vi "render.vi"(6 "Numeric":i32, 9 "origin":cluster{"left":i16, "top":i16}, 10 "new picture in":picture, 11 "map":i8[][][](array[numeric])) -> (3 "new picture out":picture)   [LabVIEW 2025]
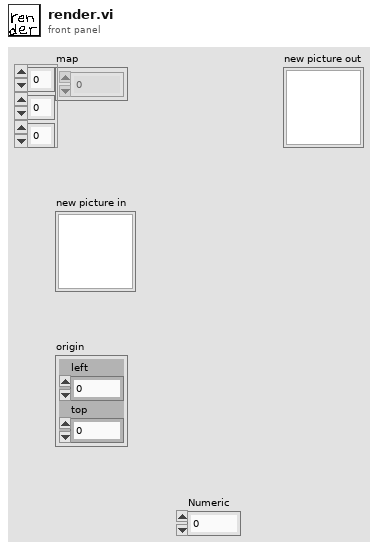
[diagram p1: front panel]
types:
  T1 = enum16{"User-specified Font", "Application Font", "System Font", "Dialog Font"}
  T2 = cluster{"Font Name:":string, "Size":i16, "Strikeout?":bool, "Italic?":bool, "Underline?":bool, "Outline?":bool, "Shadow?":bool, "Bold?":bool}
  T3 = cluster{"left":i16, "top":i16, "right":i16, "bottom":i16}
  T4 = typedef "imagedata.ctl" = cluster{"image type":i32, "image depth":i32, "image":u8[], "mask":u8[], "colors":u32[], "Rectangle":cluster{"left":i16, "top":i16, "right":i16, "bottom":i16}}
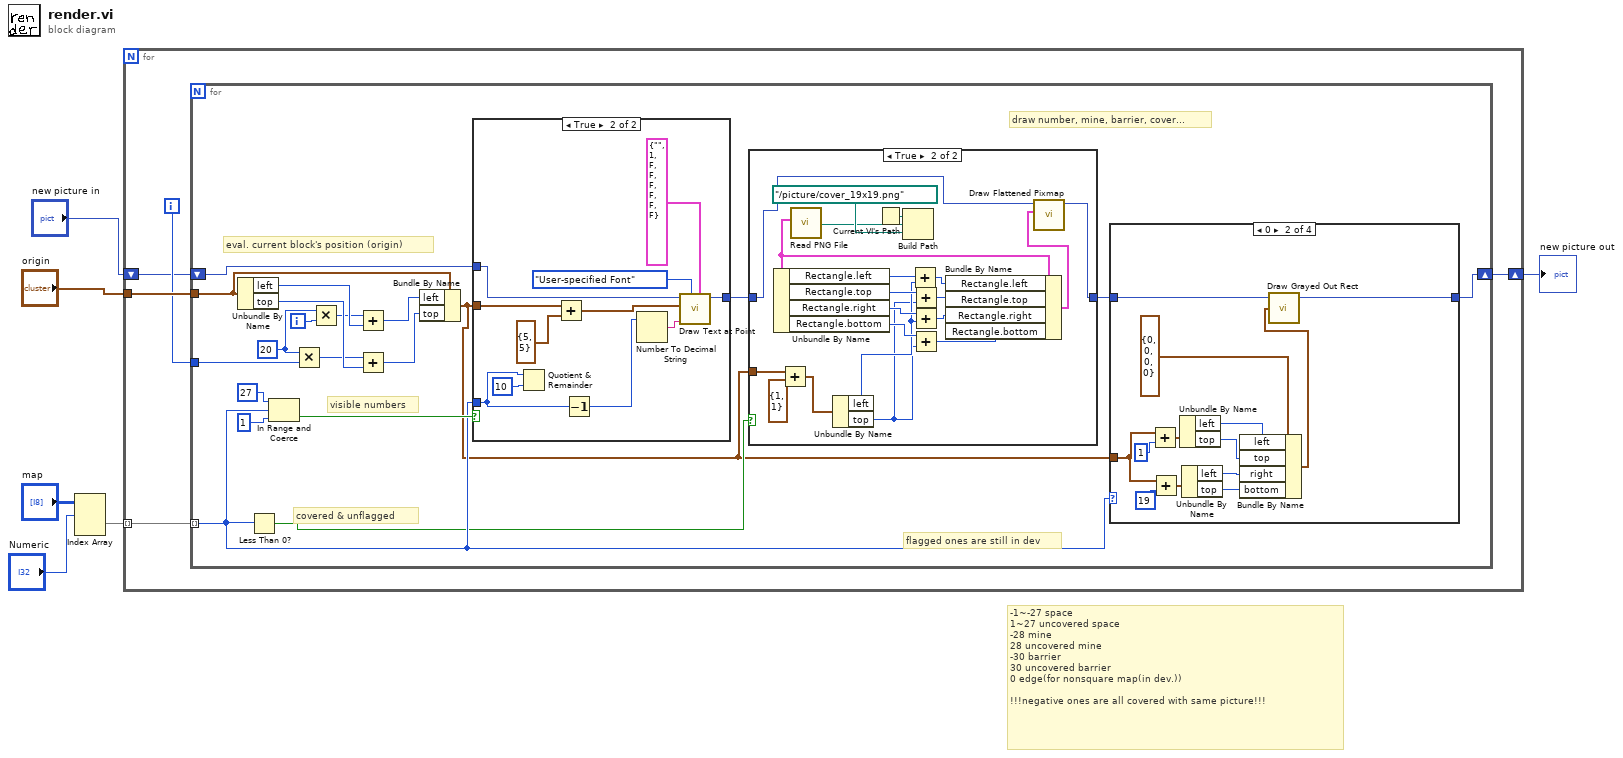
[diagram p0: block diagram]
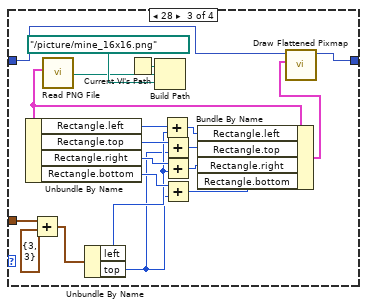
[diagram p5: hidden frame]
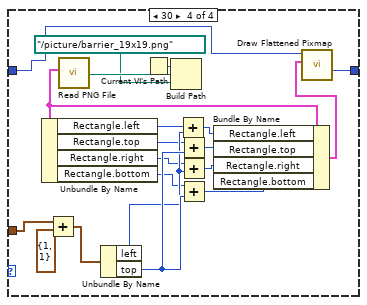
[diagram p6: hidden frame]
diagram:
  # "-1~-27 space\n1~27 uncovered space\n-28 mine\n28 uncovered mine\n-30 barrier\n30 uncovered barrier\n0 edge(for nonsquare map(in dev.))\n\n!!!negative ones are all covered with same picture!!!"
  n1 = Index Array(array="map", index (dim 0)="Numeric") -> (element=w3:i8[][])  [unwired: 2 in]
  n2 = for {
    tunnel: w3 -> [w11] mode=indexing
    tunnel: "origin" -> [w10]
    shift-right: [w7] -> w6
    shift-left: "new picture in" -> [w8]
    i -> [w9]
    n3 = for {
      tunnel: w11 -> [w14] mode=indexing
      tunnel: w10 -> [w20]
      tunnel: w9 -> [w30]
      shift-right: [w15] -> w7
      shift-left: w8 -> [w26]
      i -> [w31]
      w25 = 20 ("x")
      # "draw number, mine, barrier, cover..."
      # "flagged ones are still in dev"
      # "covered & unflagged"
      # "visible numbers"
      # "eval. current block's position (origin)"
      n4 = Unbundle By Name(w20) -> ("left"=w24:i16, "top"=w23:i16)
      n5 = Less Than 0?(x=w14) -> (x < 0?=w13:bool)
      n6 = In Range and Coerce(upper limit=i8 27, x=w14, lower limit=i8 1) -> (In Range?=w27:bool)  [unwired: 1 out]
      n7 = Multiply(x=w25, y=w30) -> (x*y=w19:i32)
      n8 = Multiply(x=w25, y=w31) -> (x*y=w18:i32)
      n9 = Add(x=w18, y=w24) -> (x+y=w22:i32)
      n10 = Add(x=w19, y=w23) -> (x+y=w21:i32)
      n11 = Bundle By Name(cluster=w20, "left"=w22, "top"=w21) -> (w12:cluster{"left":i16, "top":i16})
      n12 = case shown="True" w27 {
        tunnel: w14 -> [_ w55]
        tunnel: w12 -> [_ w58]
        tunnel: w26 -> [w53 w60]
        tunnel: [w53 w59] -> w17
        frame False {
        }
        frame True {
          n13 = Quotient & Remainder(x=w55, y=i8 10) -> ()  [unwired: 2 out]
          n14 = Add(x=w58, y=cluster{"left":i16, "top":i16} {"left"=5, "top"=5}) -> (x+y=w57:cluster{"left":i16, "top":i16})
          n15 = Decrement(x=w55) -> (x-1=w54:i8)
          n16 = Number To Decimal String(number=w54) -> (decimal integer string=w61:string)  [unwired: 1 in]
          n17 = call <vilib>:"Draw Text at Point.vi"("[user-specified font]"=T2 {"Font Name:"="", "Size"=1, "Strikeout?"=FALSE, "Italic?"=FALSE, "Underline?"=FALSE, "Outline?"=FALSE, "Shadow?"=FALSE, "Bold?"=FALSE}, "desired font(Application)"=T1."User-specified Font", "text"=w61, "origin"=w57, "picture"=w60) -> ("new picture"=w59:picture)  [unwired: 5 in, 1 out]
        }
      }
      n18 = case shown="True" w13 {
        tunnel: w17 -> [w32 w35]
        tunnel: [w32 w34] -> w16
        tunnel: w12 -> [_ w33]
        frame False {
        }
        frame True {
          n19 = Add(x=w33, y=cluster{"left":i16, "top":i16} {"left"=1, "top"=1}) -> (x+y=w36:cluster{"left":i16, "top":i16})
          n20 = Unbundle By Name(w36) -> ("left"=w45:i16, "top"=w44:i16)
          n21 = Current VI's Path() -> (path=w52:path)
          n22 = Build Path(base path=w52, name or relative path=path "../picture/cover_19x19.png") -> (appended path=w50:path)
          n23 = call <vilib>:"Read PNG File.vi"("path to PNG file"=w50) -> ("image data"=w43:T4)  [unwired: 8 in, 2 out]
          n24 = Unbundle By Name(w43) -> ("Rectangle.left"=w49:i16, "Rectangle.top"=w48:i16, "Rectangle.right"=w47:i16, "Rectangle.bottom"=w46:i16)
          n25 = Add(x=w49, y=w45) -> (x+y=w42:i16)
          n26 = Add(x=w48, y=w44) -> (x+y=w41:i16)
          n27 = Add(x=w47, y=w45) -> (x+y=w40:i16)
          n28 = Add(x=w46, y=w44) -> (x+y=w39:i16)
          n29 = Bundle By Name(cluster=w43, "Rectangle.left"=w42, "Rectangle.top"=w41, "Rectangle.right"=w40, "Rectangle.bottom"=w39) -> (w38:T4)
          n30 = call <vilib>:"Draw Flattened Pixmap.vi"("image data"=w38, "picture"=w35) -> ("new picture"=w34:picture)  [unwired: 7 in]
        }
      }
      n31 = case shown="0" w14 {
        tunnel: w16 -> [w65 w78 w83 w101]
        tunnel: [w65 w77 w82 w100] -> w15
        tunnel: w12 -> [_ w66 w81 w99]
        frame Default {
        }
        frame 0 {
          n32 = Add(x=w66, y=1) -> (x+y=w67:cluster{"left":i32, "top":i32})
          n33 = Add(x=w66, y=19) -> (x+y=w72:cluster{"left":i32, "top":i32})
          n34 = Unbundle By Name(w67) -> ("left"=w74:i32, "top"=w73:i32)
          n35 = Unbundle By Name(w72) -> ("left"=w70:i32, "top"=w71:i32)
          n36 = Bundle By Name(cluster=T3 {"left"=0, "top"=0, "right"=0, "bottom"=0} ("rect"), "left"=w74, "top"=w73, "right"=w70, "bottom"=w71) -> (w75:T3)
          n37 = call <vilib>:"Draw Grayed Out Rect.vi"("rect"=w75, "picture"=w78) -> ("new picture"=w77:picture)  [unwired: 3 in]
        }
        frame 28 {
          n38 = Add(x=w81, y=cluster{"left":i16, "top":i16} {"left"=3, "top"=3}) -> (x+y=w79:cluster{"left":i16, "top":i16})
          n39 = Unbundle By Name(w79) -> ("left"=w91:i16, "top"=w90:i16)
          n40 = Current VI's Path() -> (path=w98:path)
          n41 = Build Path(base path=w98, name or relative path=path "../picture/mine_16x16.png") -> (appended path=w96:path)
          n42 = call <vilib>:"Read PNG File.vi"("path to PNG file"=w96) -> ("image data"=w89:T4)  [unwired: 8 in, 2 out]
          n43 = Unbundle By Name(w89) -> ("Rectangle.left"=w95:i16, "Rectangle.top"=w94:i16, "Rectangle.right"=w93:i16, "Rectangle.bottom"=w92:i16)
          n44 = Add(x=w95, y=w91) -> (x+y=w88:i16)
          n45 = Add(x=w94, y=w90) -> (x+y=w87:i16)
          n46 = Add(x=w93, y=w91) -> (x+y=w86:i16)
          n47 = Add(x=w92, y=w90) -> (x+y=w85:i16)
          n48 = Bundle By Name(cluster=w89, "Rectangle.left"=w88, "Rectangle.top"=w87, "Rectangle.right"=w86, "Rectangle.bottom"=w85) -> (w84:T4)
          n49 = call <vilib>:"Draw Flattened Pixmap.vi"("image data"=w84, "picture"=w83) -> ("new picture"=w82:picture)  [unwired: 7 in]
        }
        frame 30 {
          n50 = Add(x=w99, y=cluster{"left":i16, "top":i16} {"left"=1, "top"=1}) -> (x+y=w118:cluster{"left":i16, "top":i16})
          n51 = Unbundle By Name(w118) -> ("left"=w109:i16, "top"=w110:i16)
          n52 = Current VI's Path() -> (path=w102:path)
          n53 = Build Path(base path=w102, name or relative path=path "../picture/barrier_19x19.png") -> (appended path=w104:path)
          n54 = call <vilib>:"Read PNG File.vi"("path to PNG file"=w104) -> ("image data"=w111:T4)  [unwired: 8 in, 2 out]
          n55 = Unbundle By Name(w111) -> ("Rectangle.left"=w105:i16, "Rectangle.top"=w106:i16, "Rectangle.right"=w107:i16, "Rectangle.bottom"=w108:i16)
          n56 = Add(x=w105, y=w109) -> (x+y=w112:i16)
          n57 = Add(x=w106, y=w110) -> (x+y=w113:i16)
          n58 = Add(x=w107, y=w109) -> (x+y=w114:i16)
          n59 = Add(x=w108, y=w110) -> (x+y=w115:i16)
          n60 = Bundle By Name(cluster=w111, "Rectangle.left"=w112, "Rectangle.top"=w113, "Rectangle.right"=w114, "Rectangle.bottom"=w115) -> (w116:T4)
          n61 = call <vilib>:"Draw Flattened Pixmap.vi"("image data"=w116, "picture"=w101) -> ("new picture"=w100:picture)  [unwired: 7 in]
        }
      }
    }
  }
  "new picture out" <- w6
